vi "EncoderBegin.vi"(8 "error in (no error)":errorcluster) -> (0 "error out":errorcluster)   [LabVIEW 2014]
uses:
  <vilib>/Rock Robotics/SystemInterfaces/DIO/FPGA_DIOChannel.ctl
  <vilib>/Rock Robotics/WPI/Encoder/WPI_EncoderType.ctl
  <vilib>/Rock Robotics/WPI/Counter/WPI_CounterDigitalInputToDigitalSource.vi
  Begin Cals.vi
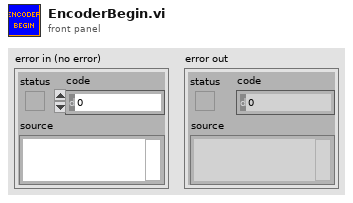
[diagram p1: front panel]
types:
  T1 = typedef "FPGA_DIOChannel.ctl" = enum8{"DIO 0", "DIO 1", "DIO 2", "DIO 3", "DIO 4", "DIO 5", "DIO 6", "DIO 7", "DIO 8", "DIO 9", "DIO MXP 0", "DIO MXP 1", "DIO MXP 2", "DIO MXP 3", "DIO MXP 4", "DIO MXP 5", "DIO MXP 6", "DIO MXP 7", "DIO MXP 8", "DIO MXP 9", "DIO MXP 10", "DIO MXP 11", "DIO MXP 12", "DIO MXP 13", "DIO MXP 14", "DIO MXP 15", "Invalid"}
  T2 = typedef "WPI_EncoderType.ctl" = enum16{"1x", "2x", "4x"}
  T3 = typedef "WPI_DigitalInputDevRef.ctl" = cluster{"DevStatus":errorcluster, "DIO Channel":T1, "Controller":T4}
  T4 = typedef "FPGA_TypedefDigitalModule.ctl" = enum16{"Controller 1"}
  T5 = typedef "FPGA_CounterEncoderSourceConvertionLVSourceType.ctl" = cluster{"DevStatus":errorcluster, "AnalogTriggerMode?":bool, "DigitalMode":cluster{"Controller":T4, "DIO Channel":T6}, "AnalogTriggerMode":cluster{"AnalogTriggerIndex":T7, "OutputType":T8}}
  T6 = typedef "FPGA_DIODigitalSourceChannel.ctl" = enum8{"DIO 0", "DIO 1", "DIO 2", "DIO 3", "DIO 4", "DIO 5", "DIO 6", "DIO 7", "DIO 8", "DIO 9", "DIO MXP 0", "DIO MXP 1", "DIO MXP 2", "DIO MXP 3", "DIO MXP 4", "DIO MXP 5", "DIO MXP 6", "DIO MXP 7", "DIO MXP 8", "DIO MXP 9", "DIO MXP 10", "DIO MXP 11", "DIO MXP 12", "DIO MXP 13", "DIO MXP 14", "DIO MXP 15", "Disabled"}
  T7 = typedef "FPGA_AnalogTriggerIndex.ctl" = enum8{"Trig 0", "Trig 1", "Trig 2", "Trig 3", "Trig 4", "Trig 5", "Trig 6", "Trig 7", "Invalid"}
  T8 = typedef "FPGA_AnalogTriggerOutType.ctl" = enum16{"InWindow", "TriggerState", "Rising", "Falling"}
  T9 = typedef "WPI_EncoderDevRef.ctl" = cluster{"DevStatus":errorcluster, "EncoderIndex":T10, "CounterIndex":T11, "DistancePerCount":dbl, "Decoding Type":T2}
  T10 = typedef "FPGA_EncoderIdx.ctl" = enum8{"Enc 0", "Enc 1", "Enc 2", "Enc 3", "Enc 4", "Enc 5", "Enc 6", "Enc 7", "Invalid"}
  T11 = typedef "FPGA_CounterCtrSystemIndex.ctl" = enum8{"Ctr 0", "Ctr 1", "Ctr 2", "Ctr 3", "Ctr 4", "Ctr 5", "Ctr 6", "Ctr 7", "Invalid"}
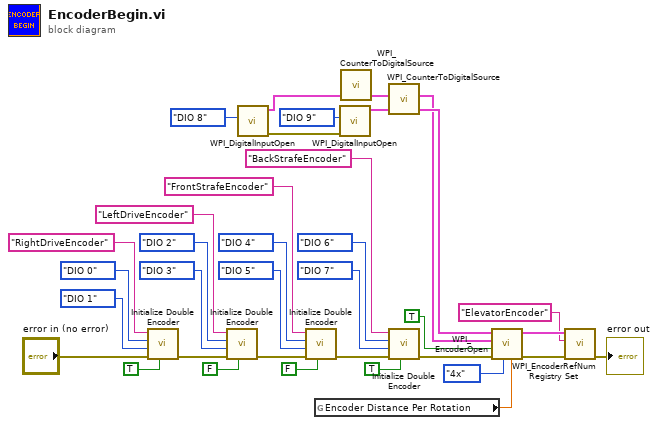
[diagram p0: block diagram]
diagram:
  n1 = call "Initialize Double Encoder.vi"("Invert Direction (False)"=TRUE, "error in (no error)"="error in (no error)", "DIO Channel 2"=FPGA_DIOChannel."DIO 1" ("DIO Channel"), "DIO Channel 1"=FPGA_DIOChannel."DIO 0" ("DIO Channel"), "refnum name"="RightDriveEncoder") -> ("error out"=w28:errorcluster)  [unwired: 6 in]
  n2 = call "Initialize Double Encoder.vi"("Invert Direction (False)"=FALSE, "error in (no error)"=w28, "DIO Channel 2"=FPGA_DIOChannel."DIO 3" ("DIO Channel"), "DIO Channel 1"=FPGA_DIOChannel."DIO 2" ("DIO Channel"), "refnum name"="LeftDriveEncoder") -> ("error out"=w25:errorcluster)  [unwired: 6 in]
  n3 = call <vilib>:"WPI_DigitalInputOpen.vi"("DIO Channel"=FPGA_DIOChannel."DIO 8") -> ("error out"=w19:errorcluster, "DigitalInputDevRef"=w15:T3)  [unwired: 9 in]
  n4 = call "Initialize Double Encoder.vi"("Invert Direction (False)"=FALSE, "error in (no error)"=w25, "DIO Channel 2"=FPGA_DIOChannel."DIO 5", "DIO Channel 1"=FPGA_DIOChannel."DIO 4" ("DIO Channel"), "refnum name"="FrontStrafeEncoder") -> ("error out"=w22:errorcluster)  [unwired: 6 in]
  n5 = global read "Begin Cals.vi" "Encoder Distance Per Rotation"() -> (w5:dbl)
  n6 = call <vilib>:"WPI_DigitalInputOpen.vi"("error in (no error)"=w19, "DIO Channel"=FPGA_DIOChannel."DIO 9") -> ("DigitalInputDevRef"=w16:T3)  [unwired: 8 in, 1 out]
  n7 = call-poly <vilib>:"WPI_CounterToDigitalSource.vi"("DigitalInputDevRef"=w15) -> ("Digital Source"=w13:T5)  [unwired: 6 in]
  n8 = call-poly <vilib>:"WPI_CounterToDigitalSource.vi"("DigitalInputDevRef"=w16) -> ("Digital Source"=w14:T5)  [unwired: 6 in]
  n9 = call "Initialize Double Encoder.vi"("Invert Direction (False)"=TRUE, "error in (no error)"=w22, "DIO Channel 2"=FPGA_DIOChannel."DIO 7", "DIO Channel 1"=FPGA_DIOChannel."DIO 6" ("DIO Channel"), "refnum name"="BackStrafeEncoder") -> ("error out"=w10:errorcluster)  [unwired: 6 in]
  n10 = call <vilib>:"WPI_EncoderOpen.vi"("DistancePerCount"=w5, "Decoding Type"=WPI_EncoderType."4x", "error in (no error)"=w10, "Invert Direction (False)"=TRUE, "BSource"=w13, "ASource"=w14) -> ("error out"=w12:errorcluster, "EncoderDevRef"=w11:T9)  [unwired: 4 in]
  n11 = call <vilib>:"WPI_EncoderRefNum Registry Set.vi"("error in (no error)"=w12, "refnum name"="ElevatorEncoder", "EncoderDevRef"=w11) -> ("error out"=→"error out":errorcluster)  [unwired: 7 in, 1 out]
